vi "load_stored_position.vi"(8 "error in (no error)":errorcluster, 11 "StageDL090409Scaffold in":refnum<class "StageDL090409Scaffold.lvclass">) -> (0 "error out":errorcluster, 3 "StageDL090409Scaffold out":refnum<class "StageDL090409Scaffold.lvclass">)   [LabVIEW 2010, in "StageDL090409Scaffold.lvclass"]
uses:
  StageDL090409Scaffold.lvclass
  stored_data_cluster.ctl
  common/classes/SpaceVector/SpaceVector/SpaceVector.lvclass
  common/classes/Image/Image/Image.lvclass
  StageDL090409Scaffold.lvclass/StageDL090409Scaffold.ctl
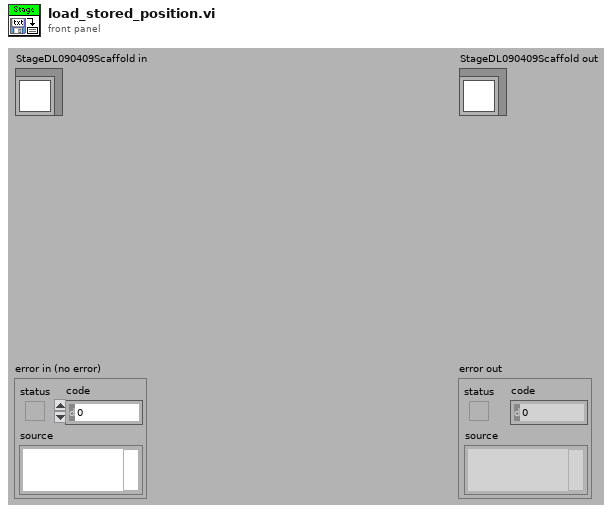
[diagram p1: front panel]
types:
  T1 = typedef "StageDL090409Scaffold.lvclass/stored_data_cluster.ctl" = cluster{"stored position":refnum<class "SpaceVector.lvclass">, "description":string, "position image":refnum<class "Image.lvclass">}
  T2 = cluster{"stored data array":T1[], "origin":refnum<class "SpaceVector.lvclass">}
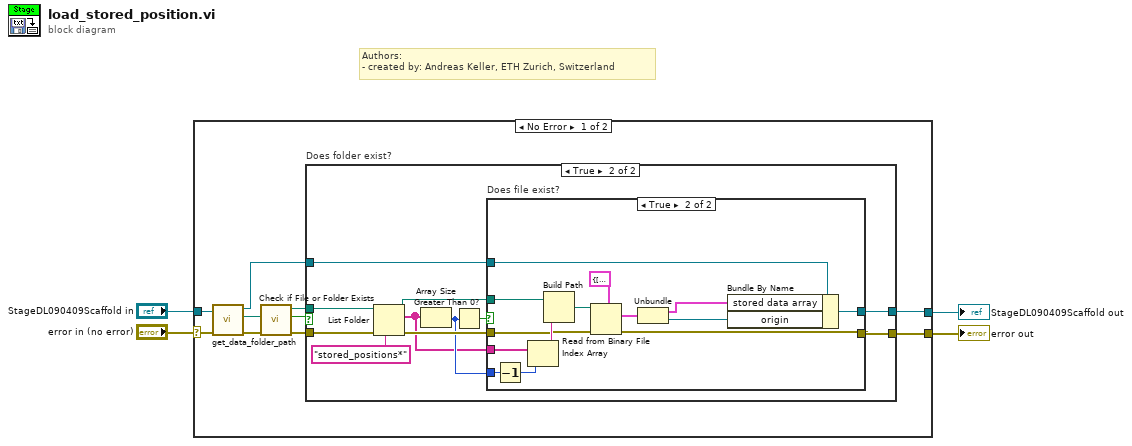
[diagram p0: block diagram]
diagram:
  # "Authors: \n- created by: Andreas Keller, ETH Zurich, Switzerland"
  n1 = case shown="No Error" "error in (no error)" {
    selector: "error in (no error)" -> [w11 w45]
    tunnel: [w7 w45] -> w3
    tunnel: [w5 w44] -> w1
    tunnel: "StageDL090409Scaffold in" -> [w8 w44]
    frame No Error {
      n2 = call-dynamic "get_data_folder_path.vi"("error in (no error)"=w11, "GenericComponent in"=w8) -> ("error out"=w10:errorcluster, "data folder path"=w9:path, "GenericComponent out"=w6:refnum<class "StageDL090409Scaffold.lvclass">)  [unwired: 7 in]
      n3 = call <vilib>:"Check if File or Folder Exists.vi"("error in (no error)"=w10, "path"=w9) -> ("error out"=w14:errorcluster, "file or folder exists?"=w12:bool, "dup path"=w13:path)  [unwired: 7 in]
      n4 = case "Does folder exist?" shown="True" w12 {
        tunnel: [w16 w19] -> w7
        tunnel: w14 -> [w16 w22]
        tunnel: w13 -> [_ w21]
        tunnel: w6 -> [w15 w18]
        tunnel: [w15 w17] -> w5
        frame False {
        }
        frame True {
          n5 = List Folder(path=w21, pattern="stored_positions*", error in=w22) -> (path out=w20:path, filenames=w23:string[], error out=w25:errorcluster)  [unwired: 1 in, 1 out]
          n6 = Array Size(array=w23) -> (size(s)=w24:i32)
          n7 = Greater Than 0?(x=w24) -> (x > 0?=w26:bool)
          n8 = case "Does file exist?" shown="True" w26 {
            tunnel: [w29 w34] -> w19
            tunnel: w25 -> [w29 w38]
            tunnel: w20 -> [_ w40]
            tunnel: w24 -> [_ w43]
            tunnel: w23 -> [_ w41]
            tunnel: w18 -> [w28 w35]
            tunnel: [w28 w33] -> w17
            frame False {
            }
            frame True {
              n9 = Decrement(x=w43) -> (x-1=w42:i32)
              n10 = Index Array(array=w41, index=w42) -> (element=w39:string)
              n11 = Build Path(base path=w40, name or relative path=w39) -> (appended path=w37:path)
              n12 = Read from Binary File(5:T2 {"stored data array"=[], "origin"=refnum} ("output cluster"), 8:w38, 11:w37) -> (0:w34:errorcluster, 2:w36:T2)  [unwired: 3 in, 2 out]
              n13 = Unbundle(w36) -> ("stored data array"=w31:T1[], "origin"=w30:refnum<class "SpaceVector.lvclass">)
              n14 = Bundle By Name(cluster=w35, "stored data array"=w31, "origin"=w30) -> (w33:refnum<class "StageDL090409Scaffold.lvclass">)
            }
          }
        }
      }
    }
    frame Error {
    }
  }
  "error out" <- w3
  "StageDL090409Scaffold out" <- w1
